vi "SMO.BasicByRef.GetPublicEventsRegistration.vi"(8 "error in (no error)":errorcluster, 11 "SMO.BasicByRef":refnum<class "SMO.BasicByRef.lvclass">) -> (0 "error out":errorcluster, 2 "SMO.BasicByRef Refnum":refnum<event-registration>, 3 "SMO.BasicByRef out":refnum<class "SMO.BasicByRef.lvclass">)   [LabVIEW 2013, in "SMO.BasicByRef.lvclass"]
doc: "---------------------------------------------------------------\nJKI State Machine Objects™\nhttp://jki.net/state-machine-objects/\nCopyright (C) 2005-2015, JKI <info@jki.net>\nALL RIGHTS RESERVEDJKI State Machine Objects (SMO) 1.0.0.5\nJKI - JKI\nCopyright (c) 2016, JKI"
uses:
  SMO.BasicByRef.lvclass
  Typedefs/PublicEvents--Cluster.ctl
  Typedefs/ValueChanged--EventData--Cluster.ctl
panel:
  # "For instructions on how to use the JKI State Machine Objects, examples and video tutorials, visit:\nhttp://jki.net/state-machine-objects/\n\nJKI State Machine Objects™\nhttp://jki.net/state-machine-objects/\nCopyright (C) 2005-2015, JKI <info@jki.net>\nALL RIGHTS RESERVED"
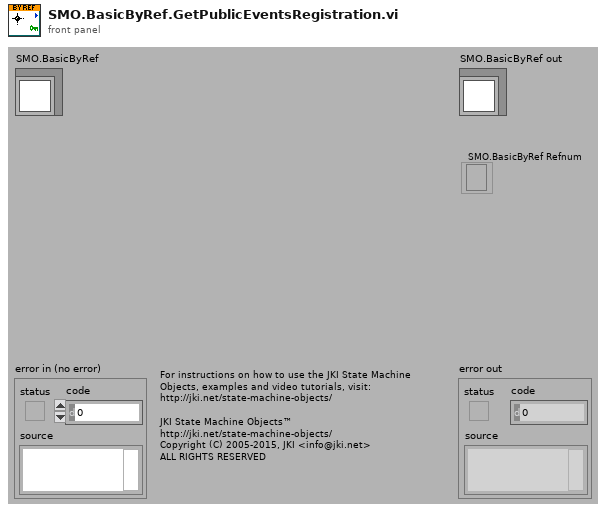
[diagram p1: front panel]
types:
  T1 = typedef "SMO.BasicByRef.lvclass/PublicEvents--Cluster.ctl" = cluster{"Value Changed":refnum<user-event>}
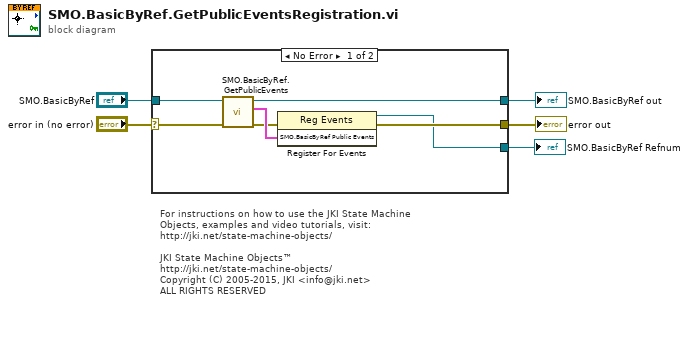
[diagram p0: block diagram]
diagram:
  # "For instructions on how to use the JKI State Machine Objects, examples and video tutorials, visit:\nhttp://jki.net/state-machine-objects/\n\nJKI State Machine Objects™\nhttp://jki.net/state-machine-objects/\nCopyright (C) 2005-2015, JKI <info@jki.net>\nALL RIGHTS RESERVED"
  n1 = case shown="No Error" "error in (no error)" {
    selector: "error in (no error)" -> [w6 w13]
    tunnel: "SMO.BasicByRef" -> [w11 w14]
    tunnel: [w9 w13] -> w4
    tunnel: [w10 w14] -> w3
    tunnel: [w8 _] -> w1
    frame No Error {
      n2 = call "SMO.BasicByRef.GetPublicEvents.vi"("error in (no error)"=w6, "SMO.BasicByRef"=w11) -> ("error out"=w7:errorcluster, "SMO.BasicByRef Public Events"=w12:T1, "SMO.BasicByRef out"=w10:refnum<class "SMO.BasicByRef.lvclass">)  [unwired: 7 in]
      n3 = register-events(error in=w7, w12) -> (reference out=w8:refnum<event-registration>, error out=w9:errorcluster)  [unwired: 1 in]
    }
    frame Error {
    }
  }
  "error out" <- w4
  "SMO.BasicByRef out" <- w3
  "SMO.BasicByRef Refnum" <- w1
